vi "HRM-Stage4-Process_main.vi"(8 "error in (no error)":errorcluster, 11 "Init cluster":T1) -> (0 "error out":errorcluster)   [LabVIEW 2020]
uses:
  initclose/HRM-Stage4-init_cluster.ctl
  initclose/HRM-stage4-config_data.ctl
  initclose/HRM-Stage4-User_events.ctl
  HRM-process-peak_detect_setting.ctl
  HRM-process-loop_cluster.ctl
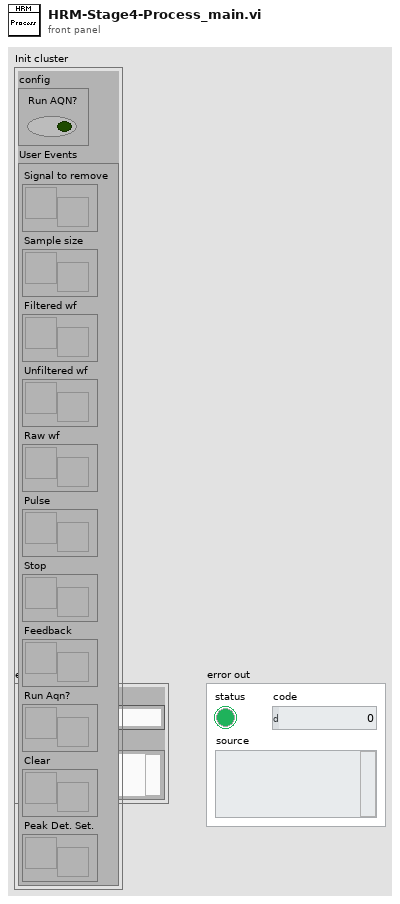
[diagram p1: front panel]
types:
  T1 = typedef "HRM-Stage4-init_cluster.ctl" = cluster{"config":T2, "User Events":T3}
  T2 = typedef "HRM-stage4-config_data.ctl" = cluster{"Run AQN?":bool}
  T3 = typedef "HRM-Stage4-User_events.ctl" = cluster{"Signal to remove":refnum<user-event>, "Sample size":refnum<user-event>, "Filtered wf":refnum<user-event>, "Unfiltered wf":refnum<user-event>, "Raw wf":refnum<user-event>, "Pulse":refnum<user-event>, "Stop":refnum<user-event>, "Feedback":refnum<user-event>, "Run Aqn?":refnum<user-event>, "Clear":refnum<user-event>, "Peak Det. Set.":refnum<user-event>}
  T4 = typedef "HRM-process-loop_cluster.ctl" = cluster{"Samples size (10)":i32, "Addition signal to remove":dbl, "Unfiltered wf":waveform(dbl), "Filtered wf":waveform(dbl), "Heart Rate":dbl, "Peak detect settings":T5, "User Events":T3}
  T5 = typedef "HRM-process-peak_detect_setting.ctl" = cluster{"Manual?":bool, "Top":dbl, "Bot":dbl}
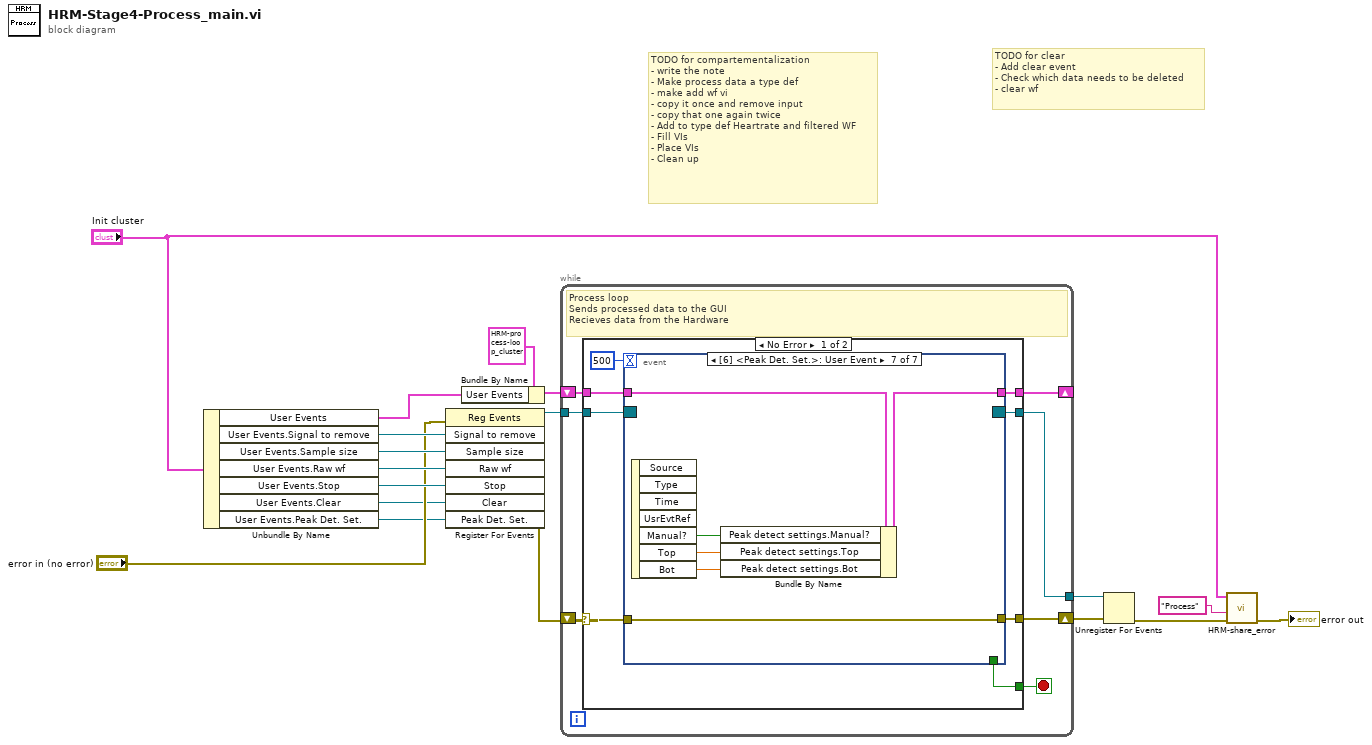
[diagram p0: block diagram]
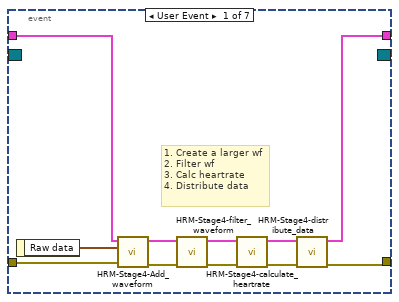
[diagram p2: hidden frame]
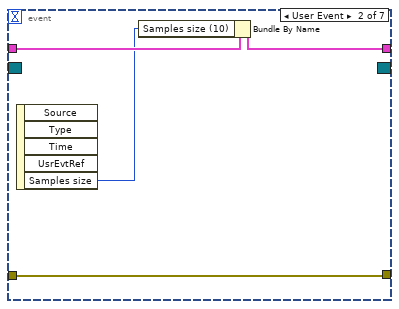
[diagram p3: hidden frame]
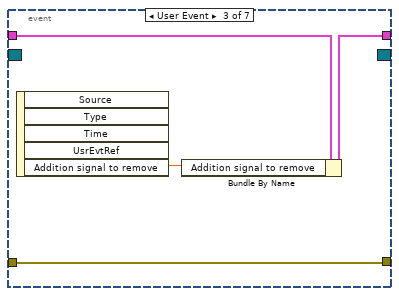
[diagram p4: hidden frame]
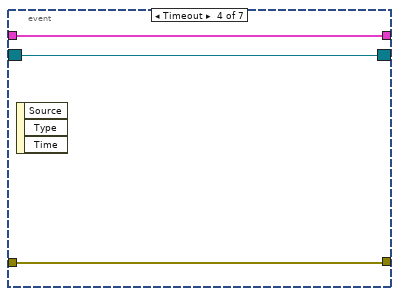
[diagram p5: hidden frame]
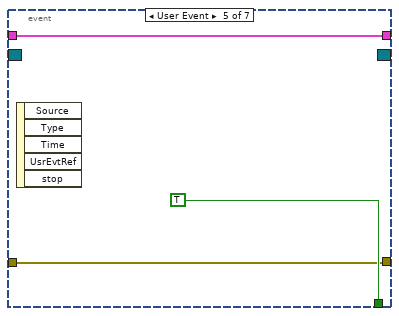
[diagram p6: hidden frame]
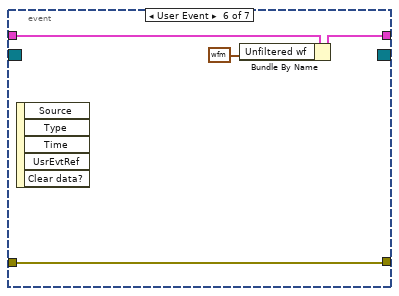
[diagram p7: hidden frame]
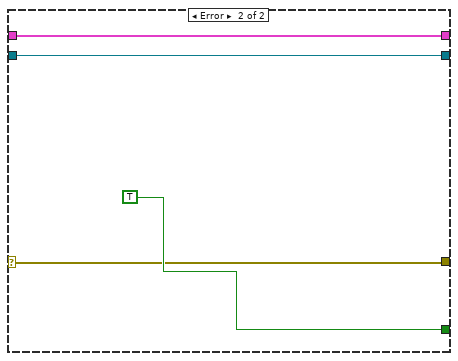
[diagram p8: hidden frame]
diagram:
  # "TODO for clear\n- Add clear event\n- Check which data needs to be deleted\n- clear wf"
  # "TODO for compartementalization\n- write the note\n- Make process data a type def\n- make add wf vi\n- copy it once and remove input \n- copy that one again twice\n- Add to type def Heartrate and filtered WF\n- Fill VIs\n- Place VIs\n- Clean up"
  n1 = Unbundle By Name("Init cluster") -> ("User Events"=w18:T3, "User Events.Signal to remove"=w16:refnum<user-event>, "User Events.Sample size"=w15:refnum<user-event>, "User Events.Raw wf"=w14:refnum<user-event>, "User Events.Stop"=w17:refnum<user-event>, "User Events.Clear"=w2:refnum<user-event>, "User Events.Peak Det. Set."=w1:refnum<user-event>)
  n2 = register-events(error in="error in (no error)", w16, w15, w14, w17, w2, w1) -> (reference out=w8:refnum<event-registration>, error out=w7:errorcluster)  [unwired: 1 in]
  n3 = Bundle By Name(cluster=T4 {"Samples size (10)"=10, "Addition signal to remove"=0.0, "Unfiltered wf"={"t0"=timestamp(0 s since 1904-01-01), "dt"=1.0, "Y"=[]}, "Filtered wf"={"t0"=timestamp(0 s since 1904-01-01), "dt"=1.0, "Y"=[]}, "Heart Rate"=0.0, "Peak detect settings"={"Manual?"=FALSE, "Top"=0.0, "Bot"=0.0}, "User Events"={"Signal to remove"=refnum, "Sample size"=refnum, "Filtered wf"=refnum, "Unfiltered wf"=refnum, "Raw wf"=refnum, "Pulse"=refnum, "Stop"=refnum, "Feedback"=refnum, "Run Aqn?"=refnum, "Clear"=refnum, "Peak Det. Set."=refnum}} ("Process data"), "User Events"=w18) -> (w10:T4)
  n4 = while {
    tunnel: w8 -> [w23]
    shift-right: [w21] -> _
    shift-left: w10 -> [w22]
    shift-right: [w20] -> w11
    shift-left: w7 -> [w24]
    tunnel: [w19] -> w12
    stop <- w25 stop-if-true
    # "Process loop\nSends processed data to the GUI\nRecieves data from the Hardware"
    n5 = case shown="No Error" w24 {
      selector: w24 -> [w30 w70]
      tunnel: [w26 TRUE ("Stop")] -> w25
      tunnel: w23 -> [w33 w69]
      tunnel: w22 -> [w32 w71]
      tunnel: [w31 w71] -> w21
      tunnel: [w29 w70] -> w20
      tunnel: [w27 w69] -> w19
      frame No Error {
        n6 = event shown="[6] <Peak Det. Set.>: User Event" {
          selector: w33 -> [_ _ _ w54 _ _ _]
          dyn-events: [_ _ _ w54 _ _ _] -> w27
          timeout: 500 -> [_ _ _ _ _ _ _]
          tunnel: w32 -> [w42 w48 w52 w55 w58 w62 w68]
          tunnel: [w34 w47 w51 w55 w58 w60 w66] -> w31
          tunnel: w30 -> [w44 w45 w49 w53 w56 w61 w67]
          tunnel: [w35 w45 w49 w53 w56 w61 w67] -> w29
          tunnel: [_ _ _ _ TRUE ("Stop") _ _] -> w26
          event User Event {
            # "1. Create a larger wf\n2. Filter wf\n3. Calc heartrate\n4. Distribute data"
            n7 = event-data() -> ("Raw data"=w43:waveform(dbl))  [unwired: 1 in]
            n8 = call "HRM-Stage4-Add_waveform.vi"("error in (no error)"=w44, "Raw wf"=w43, "Process data"=w42) -> ("error out"=w40:errorcluster, "Process data out"=w41:T4)  [unwired: 7 in]
            n9 = call "HRM-Stage4-filter_waveform.vi"("error in (no error)"=w40, "Process data"=w41) -> ("error out"=w38:errorcluster, "Process data out"=w39:T4)  [unwired: 8 in]
            n10 = call "HRM-Stage4-calculate_heartrate.vi"("error in (no error)"=w38, "Process data"=w39) -> ("error out"=w36:errorcluster, "Process data out"=w37:T4)  [unwired: 8 in]
            n11 = call "HRM-Stage4-distribute_data.vi"("error in (no error)"=w36, "Process data"=w37) -> ("error out"=w35:errorcluster, "Process data out"=w34:T4)  [unwired: 8 in]
          }
          event User Event {
            n12 = event-data() -> ("Samples size"=w46:i32)  [unwired: 1 in, 4 out]
            n13 = Bundle By Name(cluster=w48, "Samples size (10)"=w46) -> (w47:T4)
          }
          event User Event {
            n14 = event-data() -> ("Addition signal to remove"=w50:dbl)  [unwired: 1 in, 4 out]
            n15 = Bundle By Name(cluster=w52, "Addition signal to remove"=w50) -> (w51:T4)
          }
          event Timeout {
            n16 = event-data() -> ()  [unwired: 1 in, 3 out]
          }
          event User Event {
            n17 = event-data() -> ()  [unwired: 1 in, 5 out]
          }
          event User Event {
            n18 = event-data() -> ()  [unwired: 1 in, 5 out]
            n19 = Bundle By Name(cluster=w62, "Unfiltered wf"=waveform(dbl) {"t0"=timestamp(0 s since 1904-01-01), "dt"=1.0, "Y"=[]}) -> (w60:T4)
          }
          event User Event {
            n20 = event-data() -> ("Manual?"=w63:bool, "Top"=w64:dbl, "Bot"=w65:dbl)  [unwired: 1 in, 4 out]
            n21 = Bundle By Name(cluster=w68, "Peak detect settings.Manual?"=w63, "Peak detect settings.Top"=w64, "Peak detect settings.Bot"=w65) -> (w66:T4)
          }
        }
      }
      frame Error {
      }
    }
  }
  n22 = Unregister For Events(event registration refnum=w12, error in=w11) -> (error out=w6:errorcluster)
  n23 = call "HRM-share_error.vi"("error in (no error)"=w6, "module name"="Process", "Init cluster"="Init cluster") -> ("error out"=→"error out":errorcluster)  [unwired: 8 in]
